vi "State_Waiting.vi"(8 "error in (no error)":T1, 9 "Parameter":variant, 10 "Command":string, 11 "shell in":class) -> (0 "error out":T1, 2 "Debug Message":string, 3 "shell out":class)   [LabVIEW 2021, in "launcher.lvclass"]
uses:
  launcher.lvclass
  C:/Program Files (x86)/National Instruments/LabVIEW 2021/user.lib/S2 Labs/Module Framework/Modules/Base/Module.lvclass
  launcher.lvclass/launcher.ctl
  <userlib>/S2 Labs/Module Framework/Modules/Base/Module.lvclass/Module.ctl
  <userlib>/S2 Labs/CVT Toolkit/CVT.lvclass/CVT.ctl
  <userlib>/S2 Labs/Queued State Machine/TypeDefs/Queue Message.ctl
  <userlib>/S2 Labs/Queued State Machine/TypeDefs/States.ctl
  <userlib>/S2 Labs/Queued State Machine/QSM.lvclass/QSM.ctl
  4558c0cc-cebd-4e9b-9aa6-99d313716bb1.vi
  a0e8873e-df68-4f3e-a877-1e20ad01f2ca.vi
  8f6ea760-1262-4883-b350-a5244765b2be.vi
  <userlib>/S2 Labs/Module Framework/Modules/Base/Read App Start Time.vi
  <userlib>/S2 Labs/Module Framework/Modules/Base/Read App Directory.vi
  a0e8873e-df68-4f3e-a877-1e20ad01f2ca.vi/71b19a30-41bb-452f-8775-2cd3e07414b9.vi
  <userlib>/S2 Labs/Module Framework/Modules/Base/Read Module CVT.vi
  8f6ea760-1262-4883-b350-a5244765b2be.vi/a5442550-30ab-4f7c-a4e8-4e040bcf3d57.vi
  <userlib>/S2 Labs/Module Framework/Modules/Base/Read Queue.vi
  8f6ea760-1262-4883-b350-a5244765b2be.vi/77abbf80-a0d7-431e-91bd-d2268efe8bf3.vi
  8f6ea760-1262-4883-b350-a5244765b2be.vi/7a27d807-84e4-485a-8ba6-289735576614.vi
  <userlib>/S2 Labs/CVT Toolkit/Variant Functions/Write Reserved Attributes.vi
  <userlib>/S2 Labs/CVT Toolkit/Read CVT DVR.vi
  <userlib>/S2 Labs/Queued State Machine/Enqueue Element.vi
  <userlib>/S2 Labs/CVT Toolkit/Variant Functions/Write Alias Attribute.vi
  <userlib>/S2 Labs/CVT Toolkit/Variant Functions/Write Unit Attribute.vi
  <userlib>/S2 Labs/CVT Toolkit/Variant Functions/Write Type Attribute.vi
  <userlib>/S2 Labs/CVT Toolkit/Variant Functions/Write Parms Attribute.vi
  <vilib>/Utility/error.llb/Error Cluster From Error Code.vi
  <vilib>/rvi/errors/niLvFpgaAdjustHostInterfaceError.vi
  <userlib>/S2 Labs/Module Framework/Modules/Base/Trigger Logging Write.vi
  <userlib>/S2 Labs/Queued State Machine/Callback Notifier/Obtain Callback Notifier.vi
  <userlib>/S2 Labs/Queued State Machine/Callback Notifier/Release Reply Notifier.vi
  <vilib>/JDP Science/JSONtext/Variant to JSON Text.vi
  <userlib>/S2 Labs/Alarms and Events Toolkit/Alarms/Set User Event.vi
  <vilib>/rvi/interface/nirviReadWriteControl/nirviReadWriteControl.xnode
  <userlib>/S2 Labs/CVT Toolkit/CVT.lvclass
  <userlib>/S2 Labs/Queued State Machine/QSM.lvclass
  <userlib>/S2 Labs/Queued State Machine/Callback Notifier/Callback Notifier.lvclass
  <vilib>/JDP Science/JSONtext/LVClass Serializer/JSONtext LVClass Serializer.lvclass
  <userlib>/S2 Labs/Module Framework/Modules/Base/Module.lvclass
  <resource>/objmgr/nicontrollersysapi.rc
  NiFpgaLv.dll
  <vilib>/rvi/interface/Simulation/niFpgaSimulationCallBeginRW.vi
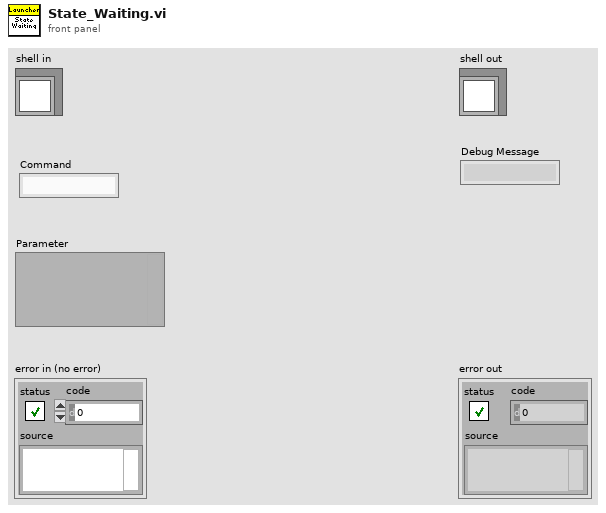
[diagram p1: front panel]
types:
  T1 = cluster{"source":string, "code":numeric, "status":boolean}
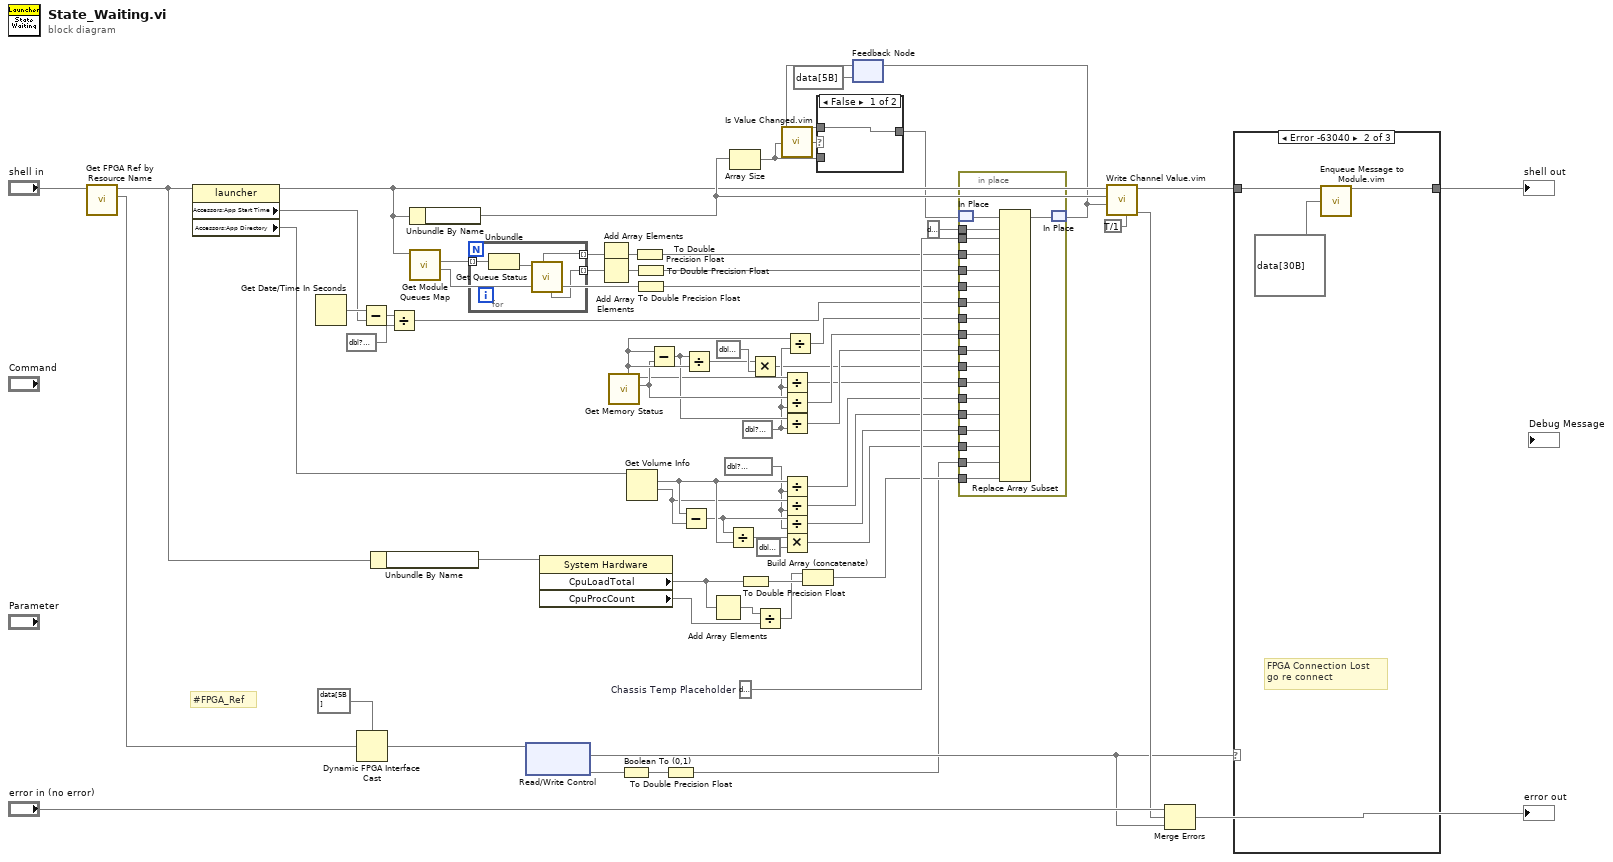
[diagram p0: block diagram]
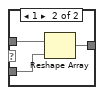
[diagram p4: hidden frame]
diagram:
  w50 = dbl? 1048576.0 ("y")
  w42 = data[9B]  # Chassis Temp Placeholder
  w48 = dbl? 1024.0 ("y")
  # "#FPGA_Ref"
  n1 = call <userlib>:"Get FPGA Ref by Resource Name.vi"(11:"shell in") -> (2:w7, 3:w8)  [unwired: 7 in, 2 out]
  n2 = property class="launcher"(reference=w8) -> (reference out=w41, "Accessors:App Start Time"=w65, "Accessors:App Directory"=w51)  [unwired: 1 in, 1 out]
  n3 = Get Date/Time In Seconds() -> (seconds since 1Jan1904=w66)
  n4 = Dynamic FPGA Interface Cast(Session In=data[5B] ("Type"), Type=w7) -> (Session Out=w5)
  n5 = Subtract(x=w66, y=w65) -> (x-y=w64)
  n6 = Unbundle By Name(w8) -> (w13)
  n7 = Divide(x=w64, y=dbl? 3600.0) -> (x/y=w31)
  n8 = Unbundle By Name(w41) -> (w44)
  n9 = call <userlib>:"Get Module Queues Map.vi"(11:w41) -> (1:w35, 2:w40)  [unwired: 7 in, 2 out]
  n10 = for {
    tunnel: w40 -> [w73] mode=indexing
    tunnel: [w71] -> w36 mode=indexing
    tunnel: [w70] -> w37 mode=indexing
    n11 = Unbundle(w73) -> (w72)  [unwired: 1 out]
    n12 = call <userlib>:"Get Queue Status.vi"(11:w72) -> (4:w71, 7:w70)  [unwired: 3 in, 6 out]
  }
  n13 = xnode "Read/Write Control"(w5) -> (w4, w3)  [unwired: 1 in, 1 out]
  n14 = property class="System Hardware"(reference=w13) -> ("CpuLoadTotal"=w16, "CpuProcCount"=w15)  [unwired: 1 in, 2 out]
  n15 = Add Array Elements(numeric array=w37) -> (sum=w39)
  n16 = Add Array Elements(numeric array=w36) -> (sum=w38)
  n17 = call <vilib>:"Get Memory Status.vi"() -> (2:w62, 3:w49, 5:w67)  [unwired: 8 in, 1 out]
  n18 = Boolean To (0,1)(Boolean=w3) -> (0, 1=w2)
  n19 = Get Volume Info(11:w51) -> (1:w52, 2:w54)  [unwired: 1 in, 4 out]
  n20 = To Double Precision Float(number=w39) -> (double precision float=w34)
  n21 = To Double Precision Float(number=w38) -> (double precision float=w33)
  n22 = To Double Precision Float(number=w35) -> (double precision float=w32)
  n23 = Subtract(x=w67, y=w62) -> (x-y=w61)
  n24 = To Double Precision Float(number=w2) -> (double precision float=w1)
  n25 = Subtract(x=w54, y=w52) -> (x-y=w53)
  n26 = Divide(x=w61, y=w67) -> (x/y=w68)
  n27 = Add Array Elements(numeric array=w16) -> (sum=w14)
  n28 = Divide(x=w53, y=w54) -> (x/y=w56)
  n29 = Array Size(array=w44) -> (size(s)=w46)
  n30 = To Double Precision Float(number=w16) -> (double precision float=w18)
  n31 = Multiply(x=w68, y=dbl? 100.0) -> (x*y=w27)
  n32 = Divide(x=w14, y=w15) -> (x/y=w17)
  n33 = call "Is Value Changed.vim"(1:w46) -> (0:w45)
  n34 = Divide(x=w49, y=w48) -> (x/y=w26)
  n35 = Divide(x=w62, y=w48) -> (x/y=w29)
  n36 = Divide(x=w61, y=w48) -> (x/y=w28)
  n37 = Divide(x=w54, y=w50) -> (x/y=w25)
  n38 = Divide(x=w52, y=w50) -> (x/y=w24)
  n39 = Divide(x=w53, y=w50) -> (x/y=w23)
  n40 = Multiply(x=w56, y=dbl? 100.0) -> (x*y=w22)
  n41 = Divide(x=w67, y=w48) -> (x/y=w30)
  n42 = Build Array (concatenate)(w17, w18) -> (w12)
  n43 = feedback #1(data[5B]) -> (w47)
  n44 = case shown="False" w45 {
    tunnel: w46 -> [_ w75]
    tunnel: [w74 w76] -> w21
    tunnel: w47 -> [w74 w77]
    frame 0 {
    }
    frame 1 {
      n45 = Reshape Array(w77, w75) -> (w76)
    }
  }
  n46 = in-place {
    in-place-border: data[5B] ("index") -> [w96]
    in-place-border: w42 -> [w95]
    in-place-border: w34 -> [w94]
    in-place-border: w33 -> [w93]
    in-place-border: w32 -> [w92]
    in-place-border: w31 -> [w91]
    in-place-border: w30 -> [w90]
    in-place-border: w29 -> [w89]
    in-place-border: w28 -> [w88]
    in-place-border: w27 -> [w87]
    in-place-border: w26 -> [w86]
    in-place-border: w25 -> [w85]
    in-place-border: w24 -> [w84]
    in-place-border: w23 -> [w83]
    in-place-border: w22 -> [w82]
    in-place-border: w12 -> [w79]
    in-place-border: w1 -> [w78]
    n47 = in-place-match #2(w21) -> (w81)
    n48 = Replace Array Subset(array=w81, new element #1=w95, index #1=w96, new element #2=w94, new element #3=w93, new element #4=w92, new element #5=w91, new element #6=w90, new element #7=w89, new element #8=w88, new element #9=w87, new element #10=w86, new element #11=w85, new element #12=w84, new element #13=w83, new element #14=w82, new element #15=w78, new element #16=w79) -> (w80)  [unwired: 15 in]
    n49 = in-place-match #2(w80) -> (w19)
  }
  n50 = feedback-in #1(w19) -> ()
  n51 = call "Write Channel Value.vim"(4:T/1 ("Trigger Logging Write? (F)"), 9:w19, 10:w44, 11:w41) -> (0:w58, 3:w11)  [unwired: 5 in, 1 out]
  n52 = Merge Errors("error in (no error)", w58, w4) -> (→"error out")
  n53 = case shown="Error -63040" w4 {
    tunnel: w11 -> [w97 w99 w101]
    tunnel: [w97 w100 w101] -> w10
    frame ..-2147483648 {
    }
    frame -63040 {
      # "FPGA Connection Lost\ngo re connect"
      n54 = call "Enqueue Message to Module.vim"(0:w99, 7:data[30B] ("Message")) -> (4:w100)  [unwired: 8 in, 5 out]
    }
    frame Default {
    }
  }
  "shell out" <- w10
